vi "_FPGA_priRFset_SaveLoad.vi"(7 "UpdPriRFsets":bool, 11 "Load nxt":bool) -> (1 "RF Set":T1={"CycleIncrement"=2000000, "Amp"=0, "Total Ticks"=20000, "Conj Ticks"=33920, "Repeat"=128}, 2 "First set?":bool, 3 "CanLoad?":bool)   [LabVIEW 2018]
uses:
  ctl/_FPGA_priRFSettings_Parameters.ctl
  ctl/_FPGA_priRFSettings_States.ctl
  <vilib>/rvi/Memory/Memory_Emulation/nirvimemoryFastEmulation.vi
  <vilib>/rvi/Memory/Memory_Emulation/nirvimemoryEmulation.vi
  <vilib>/rvi/Emulation/niFpgaEmulationIsFPGAContextNoSignature.vi
  <vilib>/rvi/DataTransferAndStorage/Container/Common/niFpgaContainerGetUniqueNameForEmu.vi
  <vilib>/rvi/Emulation/niFpgaProcessEmulError.vi
  <vilib>/rvi/Emulation/niFpgaSctlEmulationGetInTimedLoop.vi
  <vilib>/rvi/errors/nirviReportUnexpectedCaseInternalError (U32).vi
  <vilib>/rvi/errors/niFpgaSetErrorForExecOnDevCompSimple.vi
  <vilib>/rvi/eio/common/nirviEmuReportErrorAndStop.vi
  <vilib>/rvi/FIFO/Fifo_Resource/nirvififoEmulationSetSize.vi
  <vilib>/rvi/FIFO/Fifo_Resource/nirviFifoEmulationQueueMgr.vi
  <instcachedir>/0/nirviFifoEmulationQueueMgr_E5CAEC123FF24DC58D834DCA3CDAA9B5.lvgen/nirviFifoEmulationQueueMgr_E5CAEC123FF24DC58D834DCA3CDAA9B5_001.vi
  <vilib>/Utility/error.llb/Clear Errors.vi
  <vilib>/rvi/FIFO/Fifo_Resource/nirvififoEmulationCreateLock.vi
  <vilib>/rvi/FIFO/Fifo_Resource/nirvififoEmulationObtainLock.vi
  <vilib>/rvi/FIFO/Fifo_Resource/nirvififoEmulationReleaseLock.vi
  <vilib>/rvi/occurrence/nirviWaitOnOccurrenceBase.vi
  <vilib>/rvi/errors/nirviReportUnexpectedCaseInternalError.vi
  <vilib>/rvi/DataTransferAndStorage/Container/XNode/niFpgaContainer.xnode
  <vilib>/rvi/FIFO/Fifo_Resource/nirvififoEmulationRead.vi
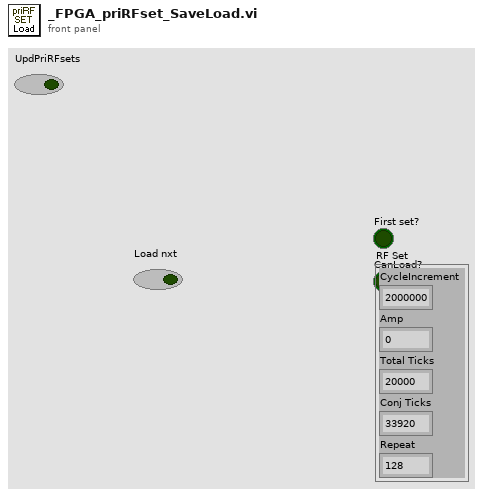
[diagram p1: front panel]
types:
  T1 = typedef "_FPGA_priRFSettings_Parameters.ctl" = cluster{"CycleIncrement":u32, "Amp":u32, "Total Ticks":u32, "Conj Ticks":u16, "Repeat":u16}
  T2 = enum16{"Idle", "Wait_for_saving_first", "Save_first_element", "Wait_for_saving", "Save_following_elements"}
  T3 = typedef "_FPGA_priRFSettings_States.ctl" = enum8{"Init", "Reading", "Placement_1", "Placement_2", "Readed"}
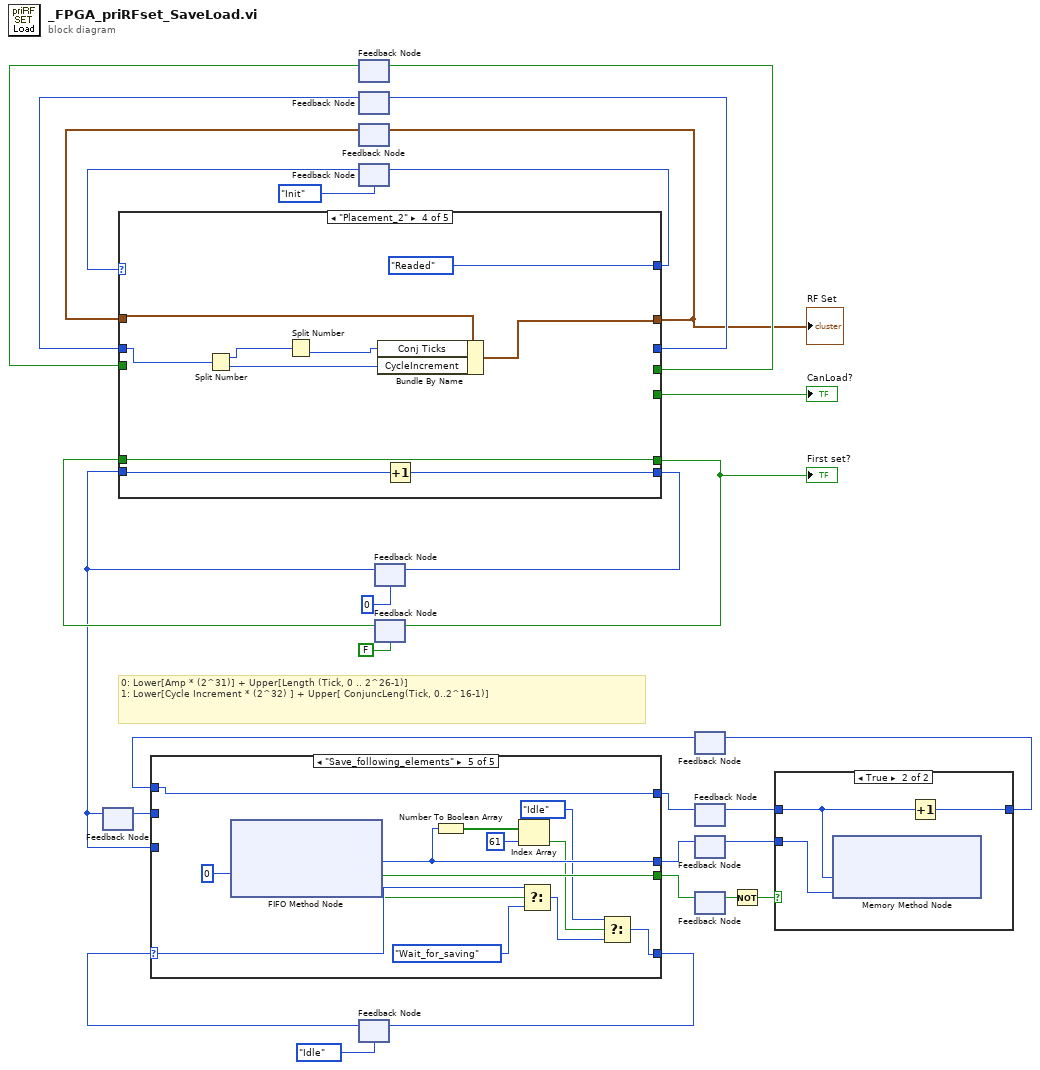
[diagram p0: block diagram]
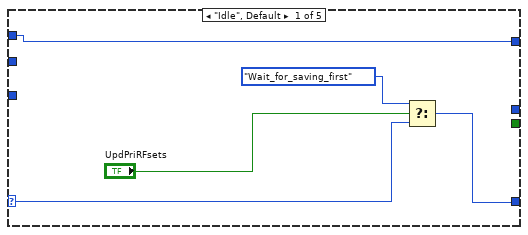
[diagram p3: hidden frame]
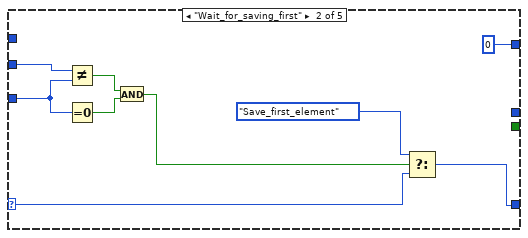
[diagram p4: hidden frame]
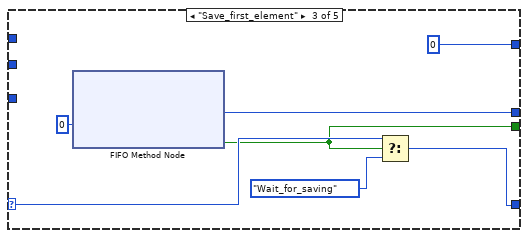
[diagram p5: hidden frame]
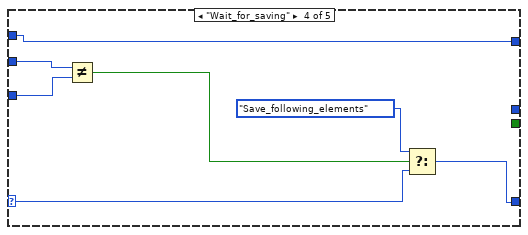
[diagram p6: hidden frame]
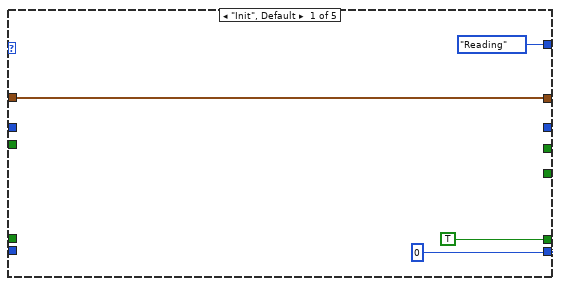
[diagram p7: hidden frame]
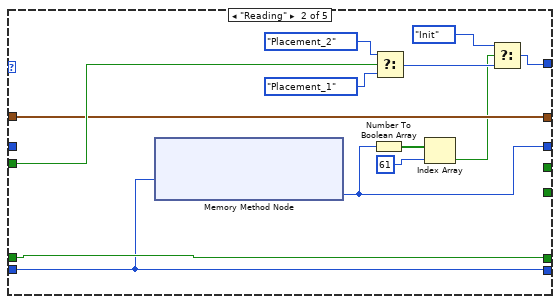
[diagram p8: hidden frame]
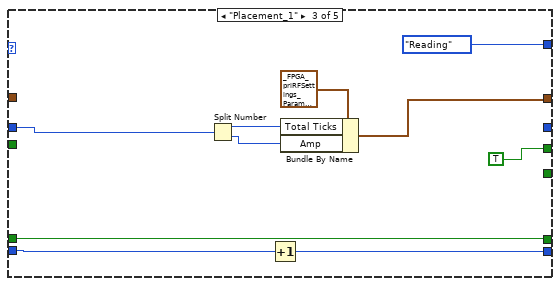
[diagram p9: hidden frame]
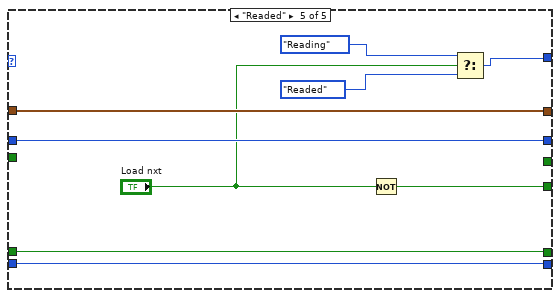
[diagram p10: hidden frame]
diagram:
  # "0: Lower[Amp * (2^31)] + Upper[Length (Tick, 0 .. 2^26-1)]\n1: Lower[Cycle Increment * (2^32) ] + Upper[ ConjuncLeng(Tick, 0..2^16-1)]"
  n1 = feedback #1() -> (w11:u8)  [unwired: 1 in]
  n2 = feedback #2() -> (w20:bool)  [unwired: 1 in]
  n3 = feedback #3() -> (w24:u64)  [unwired: 1 in]
  n4 = feedback #4() -> (w23:T1)  [unwired: 1 in]
  n5 = feedback #5(_FPGA_priRFSettings_States."Init") -> (w25:T3)
  n6 = feedback #6(T2."Idle") -> (w13:T2)
  n7 = feedback #7(u8 0) -> (w12:u8)
  n8 = feedback-in #1(w12) -> ()
  n9 = feedback #8(FALSE) -> (w17:bool)
  n10 = case shown="\"Placement_2\"" w25 {
    tunnel: [u8 0 w34 w48 w57 w75] -> w28
    tunnel: w12 -> [_ w34 w47 w58 w75]
    tunnel: [_ w39 _ _ w74] -> w27
    tunnel: [_FPGA_priRFSettings_States."Reading" w36 _FPGA_priRFSettings_States."Reading" _FPGA_priRFSettings_States."Readed" w71] -> w22
    tunnel: w24 -> [_ _ w52 w62 w74]
    tunnel: [w31 w42 w53 w65 w70] -> w15
    tunnel: w23 -> [w31 w42 _ w64 w70]
    tunnel: [_ _ TRUE _ _] -> w21
    tunnel: w20 -> [_ w45 _ _ _]
    tunnel: [_ _ _ _ w69] -> w19
    tunnel: [TRUE w43 w50 w63 w68] -> w18
    tunnel: w17 -> [_ w43 w50 w63 w68]
    frame "Init", Default {
    }
    frame "Reading" {
      n11 = xnode ("Memory Method Node")("Address"=w34) -> ("Data"=w39:u64)  [unwired: 1 in, 1 out]
      n12 = Number To Boolean Array(number=w39) -> (Boolean array=w40:bool[])
      n13 = Select(t=_FPGA_priRFSettings_States."Placement_2", s=w45, f=_FPGA_priRFSettings_States."Placement_1") -> (s? t:f=w37:T3)
      n14 = Index Array(array=w40, index=61) -> (element=w35:bool)
      n15 = Select(t=_FPGA_priRFSettings_States."Init", s=w35, f=w37) -> (s? t:f=w36:T3)
    }
    frame "Placement_1" {
      n16 = Split Number(x=w52) -> (hi(x)=w55:u32, lo(x)=w54:u32)
      n17 = Increment(x=w47) -> (x+1=w48:u8)
      n18 = Bundle By Name(cluster=T1 {"CycleIncrement"=2000000, "Amp"=0, "Total Ticks"=20000, "Conj Ticks"=33920, "Repeat"=128}, "Total Ticks"=w55, "Amp"=w54) -> (w53:T1)
    }
    frame "Placement_2" {
      n19 = Split Number(x=w62) -> (hi(x)=w61:u32, lo(x)=w59:u32)
      n20 = Split Number(x=w61) -> (lo(x)=w60:u16)  [unwired: 1 out]
      n21 = Bundle By Name(cluster=w64, "Conj Ticks"=w60, "CycleIncrement"=w59) -> (w65:T1)
      n22 = Increment(x=w58) -> (x+1=w57:u8)
    }
    frame "Readed" {
      n23 = Not(x="Load nxt") -> (.not. x?=w69:bool)
      n24 = Select(t=_FPGA_priRFSettings_States."Reading", s="Load nxt", f=_FPGA_priRFSettings_States."Readed") -> (s? t:f=w71:T3)
    }
  }
  "CanLoad?" <- w19
  "RF Set" <- w15
  "First set?" <- w18
  n25 = feedback-in #2(w21) -> ()
  n26 = feedback-in #3(w27) -> ()
  n27 = feedback-in #4(w15) -> ()
  n28 = feedback-in #5(w22) -> ()
  n29 = feedback-in #7(w28) -> ()
  n30 = feedback-in #8(w18) -> ()
  n31 = feedback #9() -> (w1:u8)  [unwired: 1 in]
  n32 = case shown="\"Save_following_elements\"" w13 {
    selector: w13 -> [w78 w84 w95 w101 w114]
    tunnel: w12 -> [_ w88 _ w102 _]
    tunnel: w11 -> [_ w89 _ w103 _]
    tunnel: [w79 w83 w94 w100 w105] -> w10
    tunnel: [_ _ w93 _ w110] -> w9
    tunnel: [_ _ w92 _ w113] -> w8
    tunnel: [w76 u8 0 u8 0 w97 w111] -> w4
    tunnel: w1 -> [w76 _ _ w97 w111]
    frame "Idle", Default {
      n33 = Select(t=T2."Wait_for_saving_first", s="UpdPriRFsets", f=w78) -> (s? t:f=w79:T2)
    }
    frame "Wait_for_saving_first" {
      n34 = Not Equal?(x=w89, y=w88) -> (x != y?=w87:bool)
      n35 = Equal To 0?(x=w88) -> (x = 0?=w86:bool)
      n36 = And(x=w87, y=w86) -> (x .and. y?=w85:bool)
      n37 = Select(t=T2."Save_first_element", s=w85, f=w84) -> (s? t:f=w83:T2)
    }
    frame "Save_first_element" {
      n38 = xnode ("FIFO Method Node")("Timeout"=0) -> ("Element"=w93:u64, "Timed Out?"=w92:bool)  [unwired: 1 in, 1 out]
      n39 = Select(t=w95, s=w92, f=T2."Wait_for_saving") -> (s? t:f=w94:T2)
    }
    frame "Wait_for_saving" {
      n40 = Not Equal?(x=w103, y=w102) -> (x != y?=w98:bool)
      n41 = Select(t=T2."Save_following_elements", s=w98, f=w101) -> (s? t:f=w100:T2)
    }
    frame "Save_following_elements" {
      n42 = xnode ("FIFO Method Node")("Timeout"=0) -> ("Element"=w110:u64, "Timed Out?"=w113:bool)  [unwired: 1 in, 1 out]
      n43 = Number To Boolean Array(number=w110) -> (Boolean array=w109:bool[])
      n44 = Index Array(array=w109, index=61) -> (element=w107:bool)
      n45 = Select(t=w114, s=w113, f=T2."Wait_for_saving") -> (s? t:f=w106:T2)
      n46 = Select(t=T2."Idle" ("f"), s=w107, f=w106) -> (s? t:f=w105:T2)
    }
  }
  n47 = feedback-in #6(w10) -> ()
  n48 = feedback #10() -> (w3:u8)  [unwired: 1 in]
  n49 = feedback-in #10(w4) -> ()
  n50 = feedback #11() -> (w5:u64)  [unwired: 1 in]
  n51 = feedback-in #11(w9) -> ()
  n52 = feedback-in #12(w8) -> ()
  n53 = feedback #12() -> (w6:bool)  [unwired: 1 in]
  n54 = Not(x=w6) -> (.not. x?=w7:bool)
  n55 = case shown="True" w7 {
    tunnel: w5 -> [_ w119]
    tunnel: w3 -> [w116 w118]
    tunnel: [w116 w117] -> w2
    frame False {
    }
    frame True {
      n56 = xnode ("Memory Method Node")("Address"=w118, "Data"=w119) -> ()  [unwired: 1 in, 1 out]
      n57 = Increment(x=w118) -> (x+1=w117:u8)
    }
  }
  n58 = feedback-in #9(w2) -> ()
